vi "command-status-ae.vi"(6 "line #":i32, 10 "ae command":T1=enum."Check last tool", 11 "tool# or drive subsystem name":string) -> (3 "Subsystem\ndone?":bool)   [LabVIEW 2017, in "labview-standard-library.lvlib" / "automode-scripting.lvlib"]
uses:
  automode-scripting.lvlib
  type-defs/command-statu-AE-control.ctl
  type-defs/tool-call-tracker.ctl
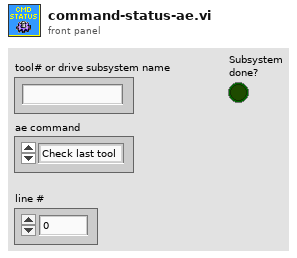
[diagram p1: front panel]
types:
  T1 = typedef "command-statu-AE-control.ctl" = enum16{"Add to sent", "Add to complete", "Check last tool", "Check specific tool"}
  T2 = typedef "tool-call-tracker.ctl" = cluster{"Tool name":string, "Count":i32, "Last line sent":i32}
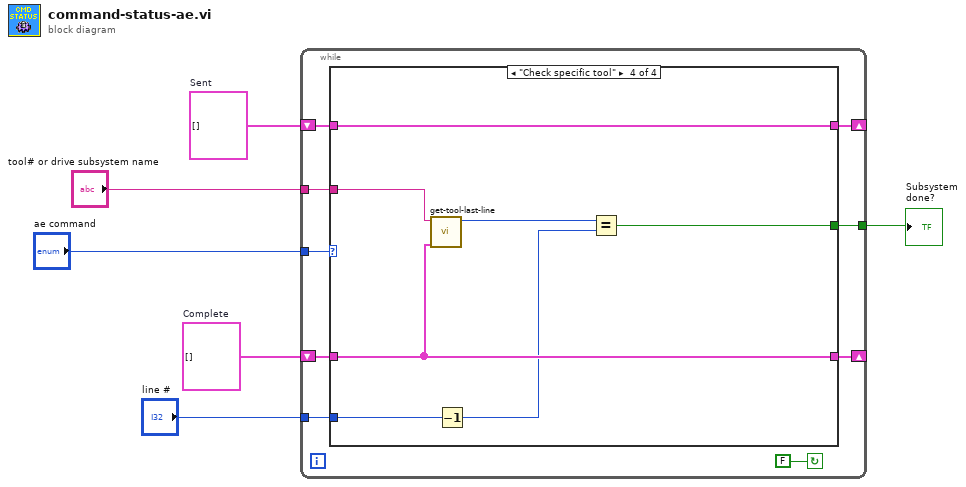
[diagram p0: block diagram]
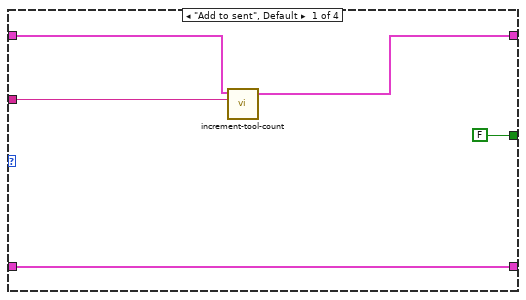
[diagram p2: hidden frame]
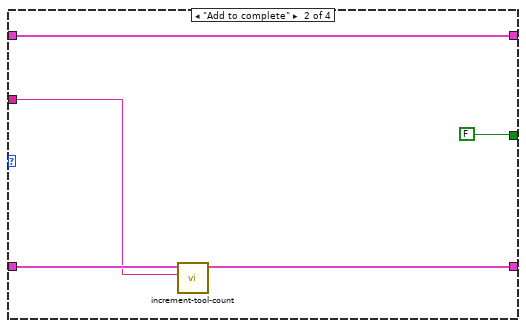
[diagram p3: hidden frame]
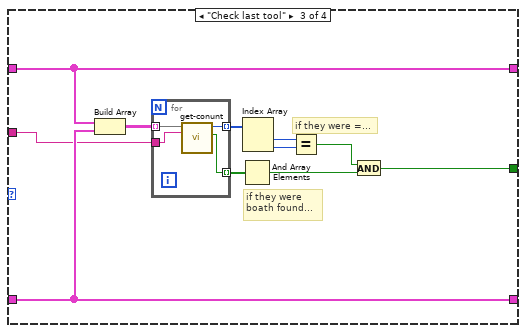
[diagram p4: hidden frame]
diagram:
  w4 = T2[] []  # Complete
  w5 = T2[] []  # Sent
  n1 = while {
    tunnel: "tool# or drive subsystem name" -> [w10]
    shift-right: [w9] -> _
    shift-left: w5 -> [w13]
    shift-right: [w11] -> _
    shift-left: w4 -> [w12]
    tunnel: "ae command" -> [w14]
    tunnel: [w8] -> w2
    tunnel: "line #" -> [w7]
    stop <- FALSE continue-if-true
    n2 = case shown="\"Check specific tool\"" w14 {
      tunnel: w13 -> [w19 w25 w36 w47]
      tunnel: [w20 w23 w35 w45] -> w11
      tunnel: w12 -> [w20 w24 w35 w45]
      tunnel: w10 -> [w18 w22 w33 w44]
      tunnel: [w17 w25 w36 w47] -> w9
      tunnel: [FALSE FALSE w26 w41] -> w8
      tunnel: w7 -> [_ _ _ w46]
      frame "Add to sent", Default {
        n3 = call "increment-tool-count.vi"("tool# or drive subsystem name"=w18, "Tool array in"=w19) -> ("Tool array out"=w17:T2[])  [unwired: 9 in]
      }
      frame "Add to complete" {
        n4 = call "increment-tool-count.vi"("tool# or drive subsystem name"=w22, "Tool array in"=w24) -> ("Tool array out"=w23:T2[])  [unwired: 9 in]
      }
      frame "Check last tool" {
        # "if they were =..."
        # "if they were\nboath found..."
        n5 = Build Array(w36, w35) -> (w34:T2[][])
        n6 = for {
          tunnel: w34 -> [w40] mode=indexing
          tunnel: w33 -> [w39]
          tunnel: [w38] -> w31 mode=indexing
          tunnel: [w37] -> w32 mode=indexing
          n7 = call "get-conunt.vi"("tool# or drive subsystem name"=w39, "Tool array in"=w40) -> ("Found?"=w37:bool, "Count"=w38:i32)  [unwired: 8 in]
        }
        n8 = And Array Elements(Boolean array=w32) -> (logical AND=w28:bool)
        n9 = Index Array(array=w31) -> (element #1=w30:i32, element #2=w29:i32)  [unwired: 2 in]
        n10 = Equal?(x=w30, y=w29) -> (x = y?=w27:bool)
        n11 = And(x=w27, y=w28) -> (x .and. y?=w26:bool)
      }
      frame "Check specific tool" {
        n12 = call "get-tool-last-line.vi"("Tool array in"=w45, "tool# or drive subsystem name"=w44) -> ("Last line sent"=w43:i32)  [unwired: 8 in, 1 out]
        n13 = Decrement(x=w46) -> (x-1=w42:i32)
        n14 = Equal?(x=w43, y=w42) -> (x = y?=w41:bool)
      }
    }
  }
  "Subsystem\ndone?" <- w2
